vi "Action Delete Curve.vi"(0 "VISA resource name":refnum<visa-resource-name>, 7 "Curve to Erase (21)":i32=21 min=21 max=60 step=1, 11 "error in (no error)":errorcluster) -> (4 "VISA resource name out":refnum<visa-resource-name>, 15 "error out":errorcluster)   [LabVIEW 2019, in "Lake Shore Cryotronics 340.lvlib"]
doc: "This VI deletes the selected user curve. Curves are not permanently updated in the curve FLASH until a Save Curve command has been issued using the LSCI 340 Save Curve to Flash.vi"
uses:
  Lake Shore Cryotronics 340.lvlib
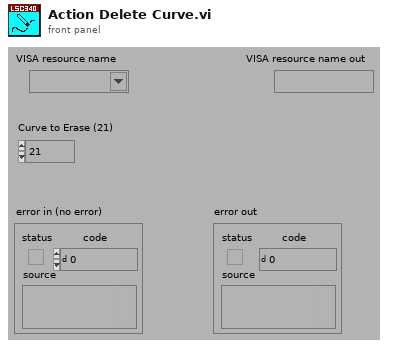
[diagram p1: front panel]
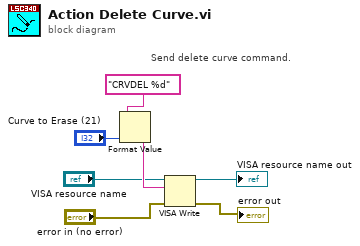
[diagram p0: block diagram]
diagram:
  # "Send delete curve command."
  n1 = Format Value(format string="CRVDEL %d", value (0)="Curve to Erase (21)") -> (output string=w5:string)  [unwired: 1 in]
  n2 = VISA Write(VISA resource name="VISA resource name", write buffer=w5, error in (no error)="error in (no error)") -> (VISA resource name out=→"VISA resource name out":refnum<visa-resource-name>, error out=→"error out":errorcluster)  [unwired: 1 out]
